vi "Display Info.vi"(7 "Layout ref":refnum<vi>, 8 "error in (no error)":errorcluster, 9 "Modify (F) /Add [T]":bool, 10 "Names in use":string[](array[string]), 11 "Device in":refnum<class "Device.lvclass">) -> (0 "error out":errorcluster, 1 "Names in use out":string[](array[string]), 2 "Changes Made?":bool, 3 "Device out":refnum<class "Device.lvclass">)   [LabVIEW 2013, in "Device.lvclass"]
uses:
  Device.lvclass
panel:
  # "This VI just sets the wiring structure.\nOpen a child override version instead!"
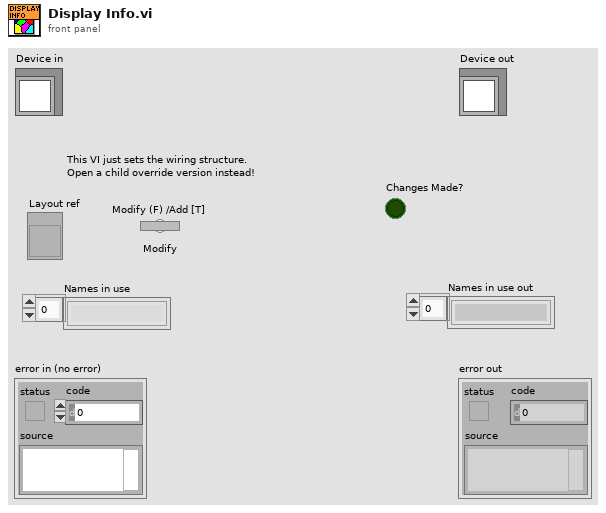
[diagram p1: front panel]
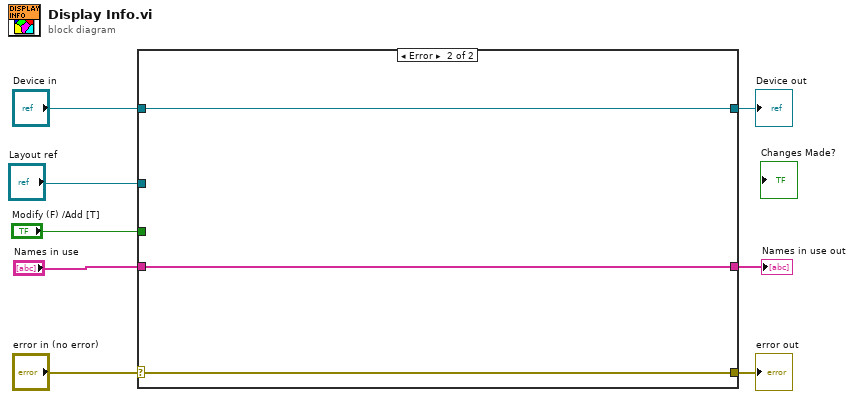
[diagram p0: block diagram]
diagram:
  n1 = case shown="Error" "error in (no error)" {
    selector: "error in (no error)" -> [w10 w14]
    tunnel: [w10 w14] -> w7
    tunnel: [w11 w13] -> w5
    tunnel: "Device in" -> [w11 w13]
    tunnel: "Layout ref" -> [_ _]
    tunnel: "Modify (F) /Add [T]" -> [_ _]
    tunnel: "Names in use" -> [w9 w12]
    tunnel: [w9 w12] -> w1
    frame No Error {
      # "Wire the error cluster across even in the \"No Error\"\ncase so that warnings get propagated."
    }
    frame Error {
    }
  }
  "error out" <- w7
  "Device out" <- w5
  "Names in use out" <- w1
